vi "jogMotor.vi"(0 "SingleAxisController in":refnum<class "_SingleAxisController.lvclass">, 2 "axis (nc - for use with multi-axis applications only)":T1, 3 "dir":T2, 5 "error in (no error)":errorcluster) -> (14 "SingleAxisController out":refnum<class "_SingleAxisController.lvclass">, 17 "success?":bool, 18 "response":string, 19 "error out":errorcluster)   [LabVIEW 2020, in "classes.lvlib" / "_SingleAxisController.lvclass"]
doc: "Produced By:\n\n<B>Kod Integrations, LLC</B>\n4835 Marianne Drive\nMount Airy, MD 21771\nhttp://www.kodintegrations.com\nemail: info@kodintegrations.com\nphone: (240) 687-1288"
uses:
  _SingleAxisController.lvclass
  _Controller.lvclass
  C:/GEECS/Developers Version/source/Device Drivers/Newmark-NSC-A/Arcus Driver 3.0.0/ArcusUsbComm/classes/Controller/_Controller.lvclass
  C:/GEECS/Developers Version/source/Device Drivers/Newmark-NSC-A/Arcus Driver 3.0.0/ArcusUsbComm/classes/SingleAxisController/_SingleAxisController.lvclass
  linear_direction.ctl
  common.lvlib
  axis.ctl
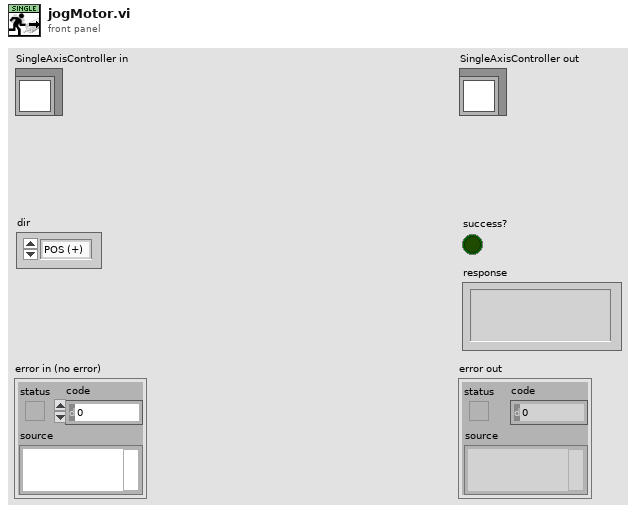
[diagram p1: front panel]
types:
  T1 = typedef "common.lvlib/axis.ctl" = enum16{"X", "Y", "Z", "U"}
  T2 = typedef "common.lvlib/linear_direction.ctl" = enum16{"POS (+)", "NEG (-)"}
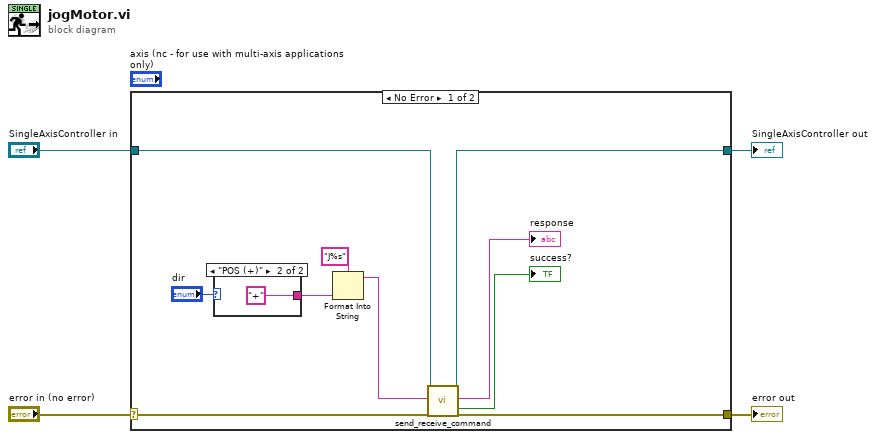
[diagram p0: block diagram]
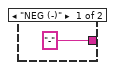
[diagram p2: hidden frame]
diagram:
  n1 = case shown="No Error" "error in (no error)" {
    selector: "error in (no error)" -> [w8 w18]
    tunnel: [w7 w18] -> w3
    tunnel: [w5 w17] -> w1
    tunnel: "SingleAxisController in" -> [w6 w17]
    frame No Error {
      n2 = case shown="\"POS (+)\"" "dir" {
        tunnel: ["-" "+"] -> w10
        frame "NEG (-)" {
        }
        frame "POS (+)" {
        }
      }
      n3 = Format Into String(format string="J%s", w10) -> (resulting string=w9:string)  [unwired: 2 in, 1 out]
      n4 = call "send_receive_command.vi"("reference (in)"=w6, "ASCII Command (in)"=w9, "error in (no error)"=w8) -> ("reference (out)"=w5:refnum<class "_SingleAxisController.lvclass">, "response (out)"=→"response":string, "success?"=→"success?":bool, "error out"=w7:errorcluster)  [unwired: 12 in, 1 out]
    }
    frame Error {
    }
  }
  "error out" <- w3
  "SingleAxisController out" <- w1
